vi "TDMS File Converter.vi"() -> ()   [LabVIEW 2023, in "GettingStarted_Common_148X_Host.lvlib"]
uses:
  GettingStarted_Common_148X_Host.lvlib
panel:
  in  "Conversion Type":string(combo)="Merge"
  out "Progress":dbl(slide) scale=0.0..1.0
  in  "Serial Input Channel":string="SI0"
  out "Error Out":errorcluster
  in  "TDMS File Directory":path
  # "Overview: Convert TDMS files between the original three file format (timestamps, sizes and data) and the newer single file format (packets). \nRequirements: FlexRIO\nInstructions: \n 1. Enter the name of the serial channel used to acquire the data.  This is used to construct the file name(s) used with the CSI-2 Getting Started Examples.\n 2. Select the conversion type:\n       Merge: Converts three files (timestamps, sizes and data) into the newer single file format (packets).\n       Split: Converts the single file format (packets) into three files (timestamps, sizes and data).\n 3. Select the directory containing the TDMS file to read and write.\n 4. Run the VI."
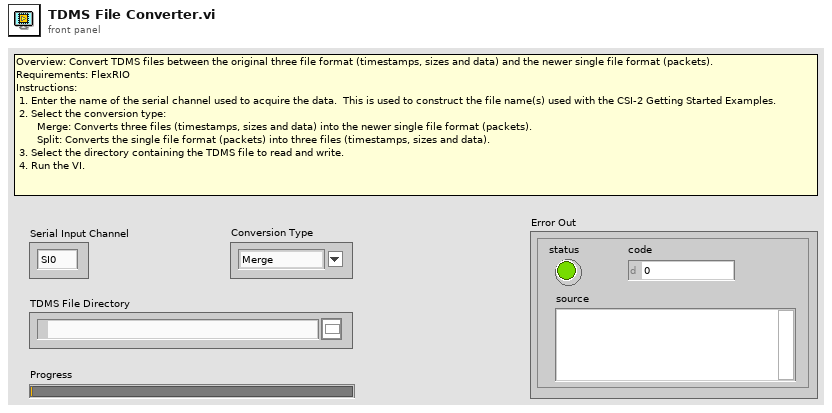
[diagram p1: front panel]
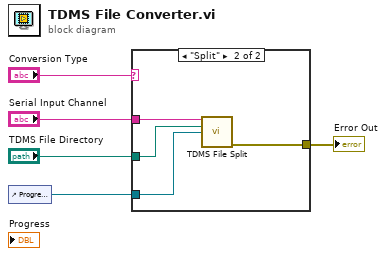
[diagram p0: block diagram]
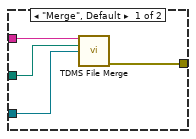
[diagram p2: hidden frame]
diagram:
  n1 = control-ref of="Progress Ref"() -> (w2:refnum<vi>)
  n2 = case shown="\"Split\"" "Conversion Type" {
    tunnel: "Serial Input Channel" -> [w9 w13]
    tunnel: "TDMS File Directory" -> [w8 w12]
    tunnel: w2 -> [w7 w11]
    tunnel: [w6 w10] -> w1
    frame "Merge", Default {
      n3 = call "TDMS File Merge.vi"("serial input channel"=w9, "tdms file directory"=w8, "progress ref"=w7) -> ("error out"=w6:errorcluster)  [unwired: 12 in]
    }
    frame "Split" {
      n4 = call "TDMS File Split.vi"("serial input channel"=w13, "tdms file directory"=w12, "progress ref"=w11) -> ("error out"=w10:errorcluster)  [unwired: 12 in]
    }
  }
  "Error Out" <- w1
